vi "Host__Main.vi"() -> ()   [LabVIEW 2018]
doc: "Main program to be run from user pc for operating pod.\nMust be run before Master__Main.vi.\n\nContains an initialization section that forces the confirmation of system run parameters and sets variables to safe values. \nThere are 4 parallel loops for: GUI updates, user events, receiving data from target, sending data via UDP (per SpaceX's requirements)"
uses:
  Globals/Host_STOP.vi
  <vilib>/Utility/error.llb/DialogType.ctl
  Master/Control/TypeDef_DigitalOuts.ctl
  Master/Control/RunTypesLibrary/RunTypeList.ctl
  Master/TypeDef_RunParameters.ctl
  Globals/Host_RUNPARAMETERS.vi
  Libraries/TypeDef_ControlTabs.ctl
  Globals/Host_UDPGLOBALS.vi
  Type_Def/Master_DataControl.ctl
  Type_Def/TypeDef FixedMotorData.ctl
  Type_Def/Type_Def Actuator Controls.ctl
  Libraries/TypeDef_CurrentState.ctl
panel:
  out "Motor Target":dbl
  out "BMS Fault":bool
  out "BMS Connection":bool
  out "Low Side (BMS)":bool
  out "High Side (BMS)":bool
  out "Motor Fault":bool
  out "Ignition Indicator":bool caption="Ignition"
  out "Speed (mph)":dbl(graph)
  in  "ReIntCAN":bool
  in  "Acc Offset":bool
  in  "Reset Navigation":bool
  out "Pump Indicator":bool caption="Pump"
  in  "Dump Valve":bool
  out "Motor Controller State":u16(ring)=1 items=["unknown"=1, "boot-up"=0, "stopped"=4, "operational"=5, "pre-operational"=127, "connection lost"=128]
  out "Motor Alive":bool
  out "Distance (ft)":dbl
  out "Connected?":bool=TRUE
  out "UDP Sent":bool
  in  "DisableWatchdog":bool
  in  "Reset to Idle":bool
  in  "Manual Brake":bool
  out "Fault?":bool=TRUE
  out "Stripe Count":dbl
  out "24V Power Indicator":bool caption="Pod\nPower"
  out "Low Side Indicator":bool caption="Low\nSide"
  in  "DisableECheck":bool
  in  "Pod Power":bool
  out "HighSide Indicator":bool caption="High\nSide"
  out "Distance bar (ft)":dbl(slide) scale=0.0..5280.0 scale format="%.3f"
  out "Current State":T1
  in  "System Parameters":bool
  in  "Extended Details":bool
  in  "Save Data":bool
  out "Release Valve Indicator":bool caption="Dump\nValve"
  out "Current Time (ms)":dbl
  out "PrechargeIndicator":bool caption="Pre-\ncharge"
  out "Brakes Indicator":bool caption="Brakes"
  in  "Stop CRIO":bool
  in  "Simulate Data":bool
  out "Clamp Indicator":bool caption="Clamp"
  out "System Check Dialogue":string
  out "x Acceleration (g)":dbl(graph)
  out "HC Table":string[][](table) caption="Table Control"
  in  "ReInt Streams":bool
  in  "Stop Host":bool
  in  "Control Tab":T2=enum."Run"
  in  "Service Button (toggle)":bool
  in  "Service Button":bool
  in  "Drive Target (service)":i16 caption="Drive Target"
  in  "Drive Mode":enum16{"velocityMode", "torqueMode", ""}(ring)
  in  "driveEnable":bool
  in  "Ignition (service)":bool
  in  "Low Side (SC)":bool caption="Low\nSide"
  in  "HighSidePermission (SC)":bool caption="High\nSide"
  in  "Brakes (SC)":bool caption="Brakes"
  in  "Clamp (SC)":bool caption="Clamp"
  in  "HighSide (SC)":bool caption="High\nSide"
  in  "Precharge (SC)":bool caption="Pre-\nCharge"
  in  "Pump (SC)":bool caption="Pump"
  in  "Ignition (SC)":bool caption="Ignition"
  in  "Drive Enable (SC)":bool caption="Drive Enable"
  in  "Drive Mode (SC)":enum16{"velocityMode", "torqueMode", ""}(ring) caption="Drive Mode"
  in  "Drive Target (SC)":i16 caption="Drive Target"
  in  "Precharge":bool
  in  "Launch":bool
  in  "Ready":bool
  in  "Ignition":bool
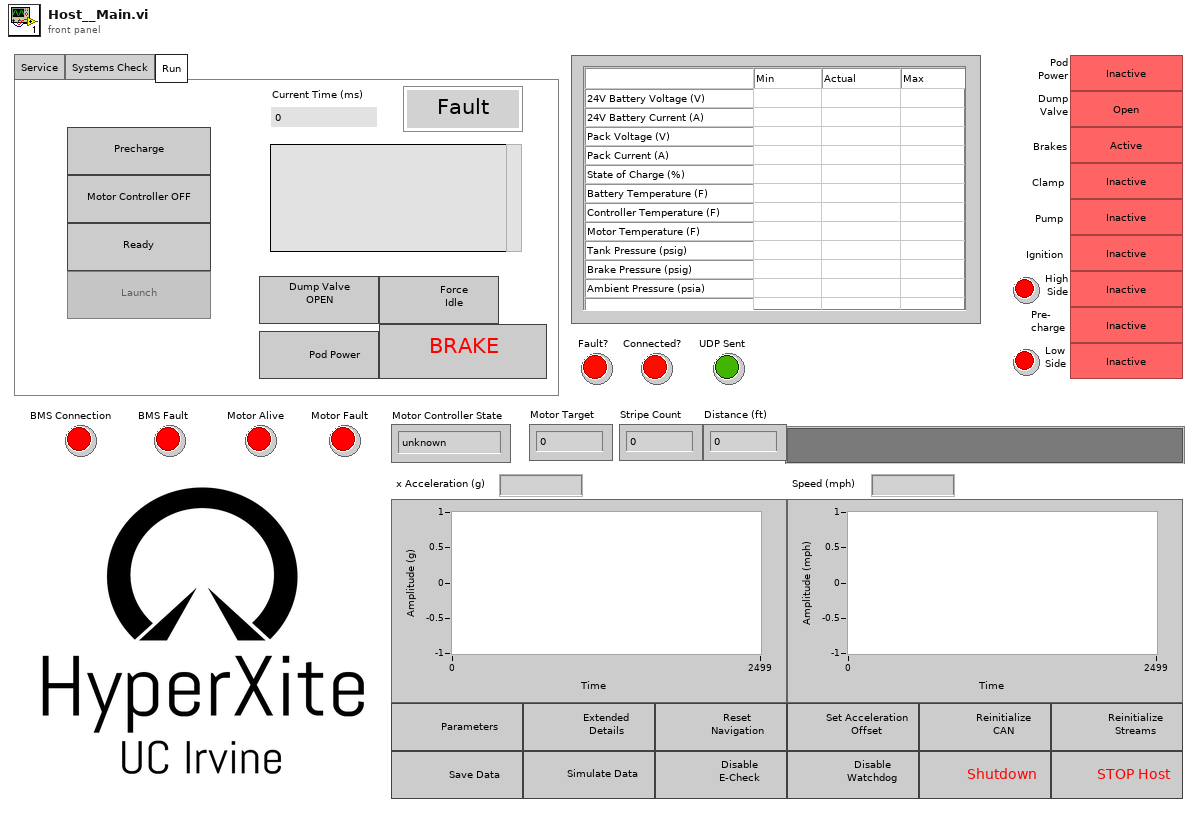
[diagram p1: front panel]
types:
  T1 = typedef "TypeDef_CurrentState.ctl" = enum16{"Fault", "Idle", "Ready", "Pushing", "Coast", "Braking"}
  T2 = typedef "TypeDef_ControlTabs.ctl" = enum32{"Service", "Systems Check", "Run"}
  T3 = typedef "DialogType.ctl" = u16
  T4 = enum8{"Enabled", "Disabled", "Disabled and Grayed Out"}
  T5 = typedef "RunTypeList.ctl" = enum16{"Full Run", "Systems Check", "Service"}
  T6 = typedef "TypeDef_RunParameters.ctl" = cluster{"Distance Threshold (ft)":dbl, "Time Threshold (s)":dbl, "Target (I16)":i16}
  T7 = typedef "TypeDef_DigitalOuts.ctl" = cluster{"Pod Power":bool, "Dump Valve":bool, "Brakes":bool, "Clamp":bool, "Pump":bool, "Ignition":bool, "DO6":bool, "DO7":bool, "HighSide":bool, "Precharge":bool, "LowSide":bool, "DO3":bool, "DO4":bool, "DO5":bool, "DO62":bool, "DO72":bool}
  T8 = typedef "Master_DataControl.ctl" = cluster{"cRIO Data":T9, "IMU Data":T10, "BMS Data":T11, "Motor Data":T13}
  T9 = typedef "TypeDef_cRIOData.ctl" = cluster{"HallEffect Right (cm)":dbl, "HallEffect Left (cm)":dbl, "Optical Sensor 1 (V)":dbl, "Optical Sensor 2 (V)":dbl, "24V Voltage  (V)":dbl, "24V Current (A)":dbl, "Contactor H1 Continuity":dbl, "Contactor L1 Continuity ":dbl, "Contactor H2 Continuity":dbl, "Contactor L2 Continuity ":dbl, "Brake PT(psig)":dbl, "Pump PT (psig)":dbl, "24V Temp   (C)":dbl, "Tank PT(psig) ":dbl, "ABS Pressure 1 (psig)":dbl, "ABS Pressure 2 (psig) ":dbl, "Displacement (ft)":dbl, "Velocity (ft/s)":dbl, "Time (ms)":dbl}
  T10 = typedef "Type_Def IMUData.ctl" = cluster{"x acceleration (g)":dbl, "Pressure (psia)":dbl, "Temperature (F)":dbl}
  T11 = typedef "TypeDef_BMSData.ctl" = cluster{"Pack 1 Max Cell\n Voltage (V)":dbl, "Pack 1 Max Cell\n ID ":dbl, "Pack 1 Min Cell \nVoltage (V)":dbl, "Pack 1 Min Cell \nID ":dbl, "Pack 1 State of Charge  (%)":dbl, "Pack 1 Average Voltage1 (V)":dbl, "Pack 1Voltage Delta (V)":dbl, "Pack 1 Current (A)":dbl, "Pack 1 Voltage (V)":dbl, "Pack 1 Max Resistance (Ohm)":dbl, "Pack 1Min Resistance (Ohm)":dbl, "Pack 1Average Resistance (Ohm)":dbl, "Pack 1Delta Resistance (Ohm)":dbl, "Pack 1 Highest Temperature(F)":dbl, "BmsStatus":T12, "Pack 2 Max Cell\n Voltage (V) ":dbl, "Pack 2 Max Cell\n ID  ":dbl, "Pack 2 Min Cell \nVoltage (V) ":dbl, "Pack 2 Min Cell \nID  ":dbl, "Pack 2 Average Voltage1 (V)":dbl, "Pack 2 Voltage Delta (V) ":dbl, "Pack 2 Current (A)":dbl, "Pack 2 Voltage (V) ":dbl, "Pack 2 State of Charge  (%) ":dbl, "Pack 2 Max Resistance (Ohm) ":dbl, "Pack 2 Min Resistance (Ohm)":dbl, "Pack 2 Average Resistance (Ohm)":dbl, "Pack 2 Delta Resistance (Ohm) ":dbl, "Pack 2 Highest Temperature(F) ":dbl}
  T12 = typedef "TypeDef_BmsStatus.ctl" = cluster{"Pack 1 Fault":bool, "Pack 1 Isolation":bool, "Pack  2 Fault":bool, "Pack 2 Isolation":bool}
  T13 = typedef "TypeDef FixedMotorData.ctl" = cluster{" Velocity (RPM)":dbl, " MotorTemp(C)":dbl, " ControlTemp(C)":dbl, " DcLinkVolt(V)":dbl, " ErrorCode":dbl, "IsAlive":bool, "motorStatus":cluster{"isReady":bool, "isOn":bool, "isOperEn":bool, "isFault":bool, "isVoltEn":bool, "targetReached":bool, "isWarning":bool}, "motorControllerState":u16}
  T14 = typedef "Type_Def Actuator Controls.ctl" = cluster{"Reverse ":bool, "Precharge Ctrl":bool, "Pump Ctrl":bool, "24 VDC Ctr":bool, "Vent Solenoid":bool, "Brake Solenoid":bool, "EMCY  Brake Solenoid":bool, "Digital Out 7B ":bool, "Forward Ctrl":bool, "Contact H1":bool, "Contact L1":bool, "Contact H2":bool, "Contact L2 ":bool, "LED RED":bool, "LED GREEN":bool, " Digital Out 7A":bool}
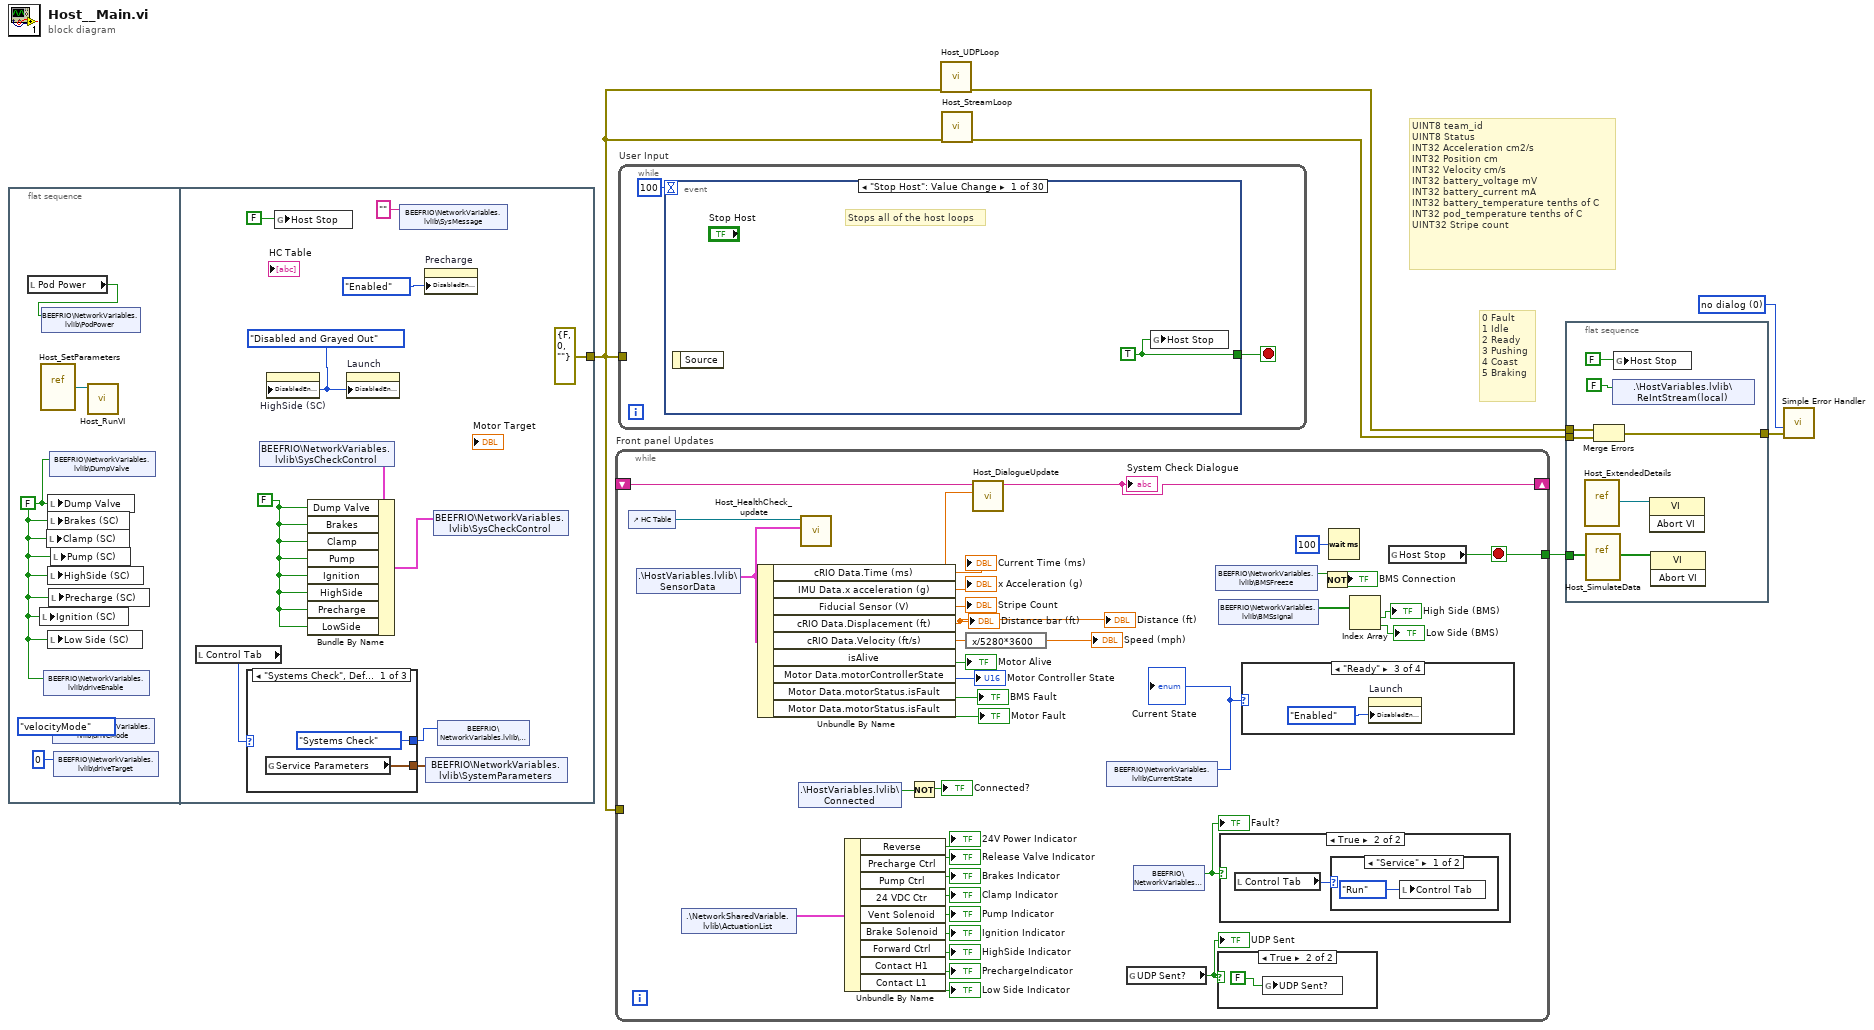
[diagram p0: block diagram]
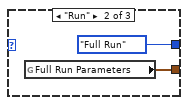
[diagram p2: hidden frame]
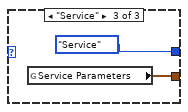
[diagram p3: hidden frame]
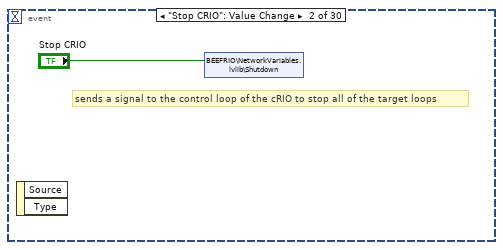
[diagram p4: hidden frame]
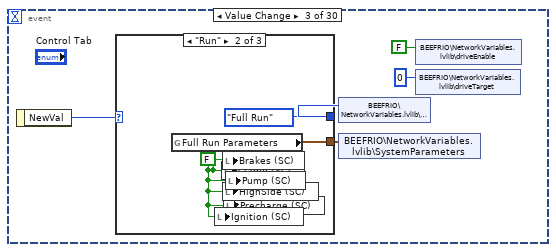
[diagram p5: hidden frame]
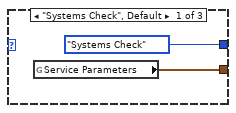
[diagram p6: hidden frame]
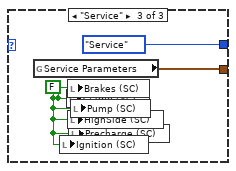
[diagram p7: hidden frame]
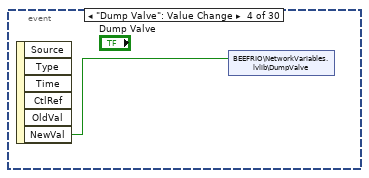
[diagram p8: hidden frame]
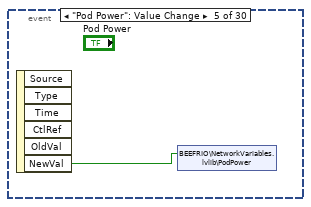
[diagram p9: hidden frame]
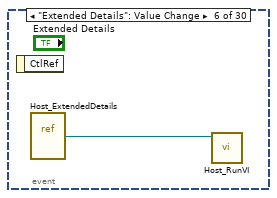
[diagram p10: hidden frame]
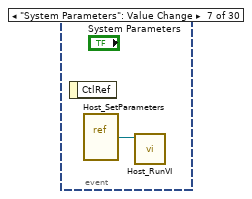
[diagram p11: hidden frame]
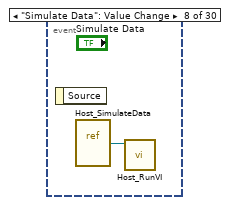
[diagram p12: hidden frame]
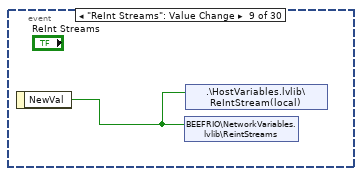
[diagram p13: hidden frame]
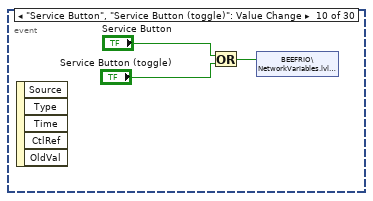
[diagram p14: hidden frame]
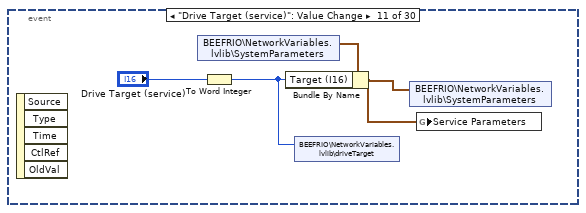
[diagram p15: hidden frame]
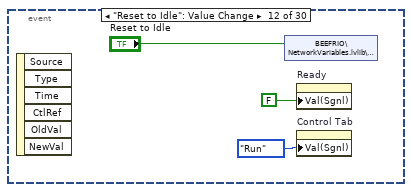
[diagram p16: hidden frame]
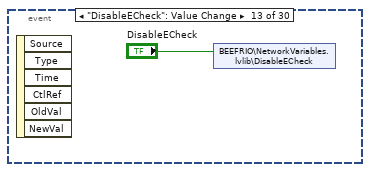
[diagram p17: hidden frame]
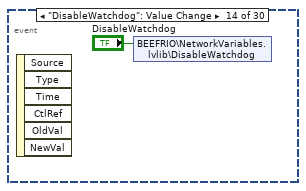
[diagram p18: hidden frame]
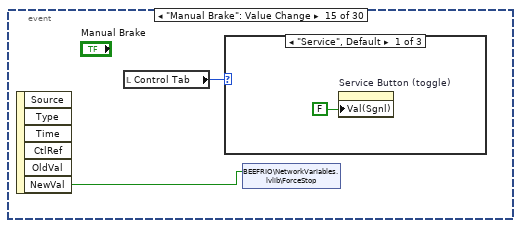
[diagram p19: hidden frame]
diagram:
  w3 = T3 0 items=["no dialog", "OK message", "continue or stop message", "OK message + warnings", "continue/stop + warnings"] ("type of dialog (OK msg:1)")
  # "0 Fault\n1 Idle\n2 Ready\n3 Pushing\n4 Coast\n5 Braking"
  # "UINT8 team_id\nUINT8 Status\nINT32 Acceleration cm2/s\nINT32 Position cm\nINT32 Velocity cm/s\nINT32 battery_voltage mV\nINT32 battery_current mA\nINT32 battery_temperature tenths of C\nINT32 pod_temperature tenths of C\nUINT32 Stripe count"
  n1 = flat-sequence {
    tunnel: [errorcluster {"status"=FALSE, "code"=0, "source"=""} ("error IO")] -> w1
    frame #0 {
      w9 = FALSE ("Dump Valve")
      n2 = local read "Pod Power"() -> (w10:bool)
      n3 = local write "Ignition (SC)"(w9) -> ()
      n4 = vi-ref "Host_SetParameters.vi"() -> (w11:refnum<vi>)
      n5 = shared-variable "BEEFRIO\\NetworkVariables.lvlib\\PodPower"(w10) -> ()  [unwired: 1 in, 1 out]
      n6 = shared-variable "BEEFRIO\\NetworkVariables.lvlib\\driveEnable"(w9) -> ()  [unwired: 1 in, 1 out]
      n7 = local write "Clamp (SC)"(w9) -> ()
      n8 = local write "Dump Valve"(w9) -> ()
      n9 = local write "Brakes (SC)"(w9) -> ()
      n10 = local write "HighSide (SC)"(w9) -> ()
      n11 = local write "Low Side (SC)"(w9) -> ()
      n12 = local write "Precharge (SC)"(w9) -> ()
      n13 = shared-variable "BEEFRIO\\NetworkVariables.lvlib\\DumpValve"(w9) -> ()  [unwired: 1 in, 1 out]
      n14 = local write "Pump (SC)"(w9) -> ()
      n15 = shared-variable "BEEFRIO\\NetworkVariables.lvlib\\driveMode"(enum16{"velocityMode", "torqueMode", ""}."velocityMode" ("driveMode")) -> ()  [unwired: 1 in, 1 out]
      n16 = shared-variable "BEEFRIO\\NetworkVariables.lvlib\\driveTarget"(i16 0 ("driveTarget")) -> ()  [unwired: 1 in, 1 out]
      n17 = call "Host_RunVI.vi"("VI in"=w11) -> ()  [unwired: 11 in]
    }
    frame #1 {
      w14 = T4."Disabled and Grayed Out" ("Disabled")
      w13 = FALSE ("Actuators.Dump Valve")
      n18 = local read "Control Tab"() -> (w20:T2)
      n19 = case shown="\"Systems Check\", Default" w20 {
        tunnel: [RunTypeList."Systems Check" ("t") RunTypeList."Full Run" ("RunType") RunTypeList."Service" ("t")] -> w19
        tunnel: [w23 w25 w28] -> w18
        frame "Systems Check", Default {
          n20 = global read "Host_RUNPARAMETERS.vi" "Service Parameters"() -> (w23:T6)
        }
        frame "Run" {
          n21 = global read "Host_RUNPARAMETERS.vi" "Full Run Parameters"() -> (w25:T6)
        }
        frame "Service" {
          n22 = global read "Host_RUNPARAMETERS.vi" "Service Parameters"() -> (w28:T6)
        }
      }
      n23 = shared-variable "BEEFRIO\\NetworkVariables.lvlib\\SysCheckControl"() -> (w17:T7)  [unwired: 1 in, 1 out]
      n24 = property on="HighSide (SC)" class="Bool (strict)"("DisabledEnum"=w14) -> ()  [unwired: 2 in, 2 out]
      n25 = global write "Host_STOP.vi" "Host Stop"(FALSE ("StopControl")) -> ()
      n26 = Bundle By Name(cluster=w17, "Dump Valve"=w13, "Brakes"=w13, "Clamp"=w13, "Pump"=w13, "Ignition"=w13, "HighSide"=w13, "Precharge"=w13, "LowSide"=w13) -> (w16:T7)
      n27 = property on="Launch" class="Bool"("DisabledEnum"=w14) -> ()  [unwired: 2 in, 2 out]
      n28 = shared-variable "BEEFRIO\\NetworkVariables.lvlib\\SysMessage"("" ("SysMessage")) -> ()  [unwired: 1 in, 1 out]
      n29 = property on="Precharge" class="Bool"("DisabledEnum"=T4."Enabled" ("Disabled")) -> ()  [unwired: 2 in, 2 out]
      n30 = shared-variable "BEEFRIO\\NetworkVariables.lvlib\\SystemParameters"(w18) -> ()  [unwired: 1 in, 1 out]
      n31 = shared-variable "BEEFRIO\\NetworkVariables.lvlib\\SysCheckControl"(w16) -> ()  [unwired: 1 in, 1 out]
      n32 = shared-variable "BEEFRIO\\NetworkVariables.lvlib\\RunType"(w19) -> ()  [unwired: 1 in, 1 out]
    }
  }
  n33 = while "Front panel Updates" {
    tunnel: [w63] -> w5
    shift-right: [w61] -> _
    shift-left: _ -> [w62]
    tunnel: w1 -> [_]
    stop <- w63 stop-if-true
    n34 = control-ref of="HC Table"() -> (w59:refnum<vi>)
    n35 = shared-variable ".\\HostVariables.lvlib\\SensorData"() -> (w58:T8)  [unwired: 1 in, 1 out]
    n36 = shared-variable ".\\NetworkSharedVariable.lvlib\\ActuationList"() -> (w60:T14)  [unwired: 1 in, 1 out]
    n37 = Unbundle By Name(w58) -> ("cRIO Data.Time (ms)"=w55:dbl, "IMU Data.x acceleration (g)"=→"x Acceleration (g)":dbl, "Fiducial Sensor (V)"=→"Stripe Count":dbl, "cRIO Data.Displacement (ft)"=→"Distance bar (ft)" →"Distance (ft)":dbl, "cRIO Data.Velocity (ft/s)"=w51:dbl, "isAlive"=→"Motor Alive":bool, "Motor Data.motorControllerState"=→"Motor Controller State":u16, "Motor Data.motorStatus.isFault"=→"BMS Fault":bool, "Motor Data.motorStatus.isFault"=→"Motor Fault":bool)
    "Current Time (ms)" <- w55
    n38 = shared-variable ".\\HostVariables.lvlib\\Connected"() -> (w53:bool)  [unwired: 1 in, 1 out]
    n39 = call "Host_HealthCheck_update.vi"("reference in"=w59, "input cluster"=w58) -> ()  [unwired: 9 in]
    n40 = Unbundle By Name(w60) -> ("Reverse"=→"24V Power Indicator":bool, "Precharge Ctrl"=→"Release Valve Indicator":bool, "Pump Ctrl"=→"Brakes Indicator":bool, "24 VDC Ctr"=→"Clamp Indicator":bool, "Vent Solenoid"=→"Pump Indicator":bool, "Brake Solenoid"=→"Ignition Indicator":bool, "Forward Ctrl"=→"HighSide Indicator":bool, "Contact H1"=→"PrechargeIndicator":bool, "Contact L1"=→"Low Side Indicator":bool)
    n41 = Not(x=w53) -> (.not. x?=→"Connected?":bool)
    n42 = expression code="x/5280*3600"(w51) -> (→"Speed (mph)":dbl)
    n43 = call "Host_DialogueUpdate.vi"("Time in"=w55, "String in"=w62) -> ("String out"=w61:string)  [unwired: 9 in]
    "System Check Dialogue" <- w61
    n44 = shared-variable "BEEFRIO\\NetworkVariables.lvlib\\CurrentState"() -> (w57:T1)  [unwired: 1 in, 1 out]
    "Current State" <- w57
    n45 = global read "Host_UDPGLOBALS.vi" "UDP Sent?"() -> (w49:bool)
    "UDP Sent" <- w49
    n46 = shared-variable "BEEFRIO\\NetworkVariables.lvlib\\Fault"() -> (w46:bool)  [unwired: 1 in, 1 out]
    "Fault?" <- w46
    n47 = shared-variable "BEEFRIO\\NetworkVariables.lvlib\\BMSFreeze"() -> (w34:bool)  [unwired: 1 in, 1 out]
    n48 = case shown="True" w49 {
      frame False {
      }
      frame True {
        n49 = global write "Host_UDPGLOBALS.vi" "UDP Sent?"(FALSE ("UDPSent?")) -> ()
      }
    }
    n50 = shared-variable "BEEFRIO\\NetworkVariables.lvlib\\BMSsignal"() -> (w35:bool[])  [unwired: 1 in, 1 out]
    n51 = case shown="True" w46 {
      frame False {
      }
      frame True {
        n52 = local read "Control Tab"() -> (w65:T2)
        n53 = case shown="\"Service\"" w65 {
          frame "Service" {
            n54 = local write "Control Tab"(TypeDef_ControlTabs."Run" ("Control Tab")) -> ()
          }
          frame Default {
          }
        }
      }
    }
    n55 = case shown="\"Ready\"" w57 {
      frame Default {
      }
      frame "Idle" {
        n56 = property on="Launch" class="Bool"("DisabledEnum"=T4."Disabled and Grayed Out" ("Disabled")) -> ()  [unwired: 2 in, 2 out]
      }
      frame "Ready" {
        n57 = property on="Launch" class="Bool"("DisabledEnum"=T4."Enabled" ("Disabled")) -> ()  [unwired: 2 in, 2 out]
      }
      frame "Pushing" {
        n58 = property on="Launch" class="Bool"("DisabledEnum"=T4."Disabled and Grayed Out" ("Disabled")) -> ()  [unwired: 2 in, 2 out]
      }
    }
    n59 = Not(x=w34) -> (.not. x?=→"BMS Connection":bool)
    n60 = Wait (ms)(milliseconds to wait=u32 100) -> ()  [unwired: 1 out]
    n61 = Index Array(array=w35) -> (element #1=→"High Side (BMS)":bool, element #2=→"Low Side (BMS)":bool)  [unwired: 2 in]
    n62 = global read "Host_STOP.vi" "Host Stop"() -> (w63:bool)
  }
  n63 = while "User Input" {
    tunnel: w1 -> [_]
    stop <- w72 stop-if-true
    n64 = event shown="[0] \"Stop Host\": Value Change" {
      selector: _ -> [_ _ _ _ _ _ _ _ _ _ _ _ _ _ _ _ _ _ _ _ _ _ _ _ _ _ _ _ _ _]
      dyn-events: _ -> [_ _ _ _ _ _ _ _ _ _ _ _ _ _ _ _ _ _ _ _ _ _ _ _ _ _ _ _ _ _]
      timeout: 100 -> [_ _ _ _ _ _ _ _ _ _ _ _ _ _ _ _ _ _ _ _ _ _ _ _ _ _ _ _ _ _]
      tunnel: [w73 _ _ _ _ _ _ _ _ _ _ _ _ _ _ _ FALSE ("element") FALSE ("element") FALSE ("element") _ _ _ _ _ _ _ _ _ _ _] -> w72
      event "Stop Host": Value Change {
        w73 = TRUE ("element")
        # "Stops all of the host loops"
        n65 = event-data() -> ()  [unwired: 1 in, 1 out]
        n66 = global write "Host_STOP.vi" "Host Stop"(w73) -> ()
      }
      event "Stop CRIO": Value Change {
        # "sends a signal to the control loop of the cRIO to stop all of the target loops"
        n67 = event-data() -> ()  [unwired: 1 in, 2 out]
        n68 = shared-variable "BEEFRIO\\NetworkVariables.lvlib\\Shutdown"("Stop CRIO") -> ()  [unwired: 1 in, 1 out]
      }
      event Value Change {
        n69 = event-data() -> ("NewVal"=w78:T2)  [unwired: 1 in]
        n70 = case shown="\"Run\"" w78 {
          tunnel: [RunTypeList."Systems Check" ("t") RunTypeList."Full Run" ("RunType") RunTypeList."Service" ("t")] -> w79
          tunnel: [w80 w83 w86] -> w77
          frame "Systems Check", Default {
            n71 = global read "Host_RUNPARAMETERS.vi" "Service Parameters"() -> (w80:T6)
          }
          frame "Run" {
            w82 = FALSE ("Dump Valve")
            n72 = global read "Host_RUNPARAMETERS.vi" "Full Run Parameters"() -> (w83:T6)
            n73 = local write "Ignition (SC)"(w82) -> ()
            n74 = local write "Clamp (SC)"(w82) -> ()
            n75 = local write "Brakes (SC)"(w82) -> ()
            n76 = local write "HighSide (SC)"(w82) -> ()
            n77 = local write "Precharge (SC)"(w82) -> ()
            n78 = local write "Pump (SC)"(w82) -> ()
          }
          frame "Service" {
            w85 = FALSE ("Dump Valve")
            n79 = global read "Host_RUNPARAMETERS.vi" "Service Parameters"() -> (w86:T6)
            n80 = local write "Ignition (SC)"(w85) -> ()
            n81 = local write "Clamp (SC)"(w85) -> ()
            n82 = local write "Brakes (SC)"(w85) -> ()
            n83 = local write "HighSide (SC)"(w85) -> ()
            n84 = local write "Precharge (SC)"(w85) -> ()
            n85 = local write "Pump (SC)"(w85) -> ()
          }
        }
        n86 = shared-variable "BEEFRIO\\NetworkVariables.lvlib\\RunType"(w79) -> ()  [unwired: 1 in, 1 out]
        n87 = shared-variable "BEEFRIO\\NetworkVariables.lvlib\\SystemParameters"(w77) -> ()  [unwired: 1 in, 1 out]
        n88 = shared-variable "BEEFRIO\\NetworkVariables.lvlib\\driveEnable"(FALSE ("driveEnable")) -> ()  [unwired: 1 in, 1 out]
        n89 = shared-variable "BEEFRIO\\NetworkVariables.lvlib\\driveTarget"(i16 0 ("driveTarget")) -> ()  [unwired: 1 in, 1 out]
      }
      event "Dump Valve": Value Change {
        n90 = event-data() -> ("NewVal"=w88:bool)  [unwired: 1 in, 5 out]
        n91 = shared-variable "BEEFRIO\\NetworkVariables.lvlib\\DumpValve"(w88) -> ()  [unwired: 1 in, 1 out]
      }
      event "Pod Power": Value Change {
        n92 = event-data() -> ("NewVal"=w89:bool)  [unwired: 1 in, 5 out]
        n93 = shared-variable "BEEFRIO\\NetworkVariables.lvlib\\PodPower"(w89) -> ()  [unwired: 1 in, 1 out]
      }
      event "Extended Details": Value Change {
        n94 = event-data() -> ()  [unwired: 1 in, 1 out]
        n95 = vi-ref "Host_ExtendedDetails.vi"() -> (w90:refnum<vi>)
        n96 = call "Host_RunVI.vi"("VI in"=w90) -> ()  [unwired: 11 in]
      }
      event "System Parameters": Value Change {
        n97 = event-data() -> ()  [unwired: 1 in, 1 out]
        n98 = vi-ref "Host_SetParameters.vi"() -> (w91:refnum<vi>)
        n99 = call "Host_RunVI.vi"("VI in"=w91) -> ()  [unwired: 11 in]
      }
      event "Simulate Data": Value Change {
        n100 = event-data() -> ()  [unwired: 1 in, 1 out]
        n101 = vi-ref "Host_SimulateData.vi"() -> (w92:refnum<vi>)
        n102 = call "Host_RunVI.vi"("VI in"=w92) -> ()  [unwired: 11 in]
      }
      event "ReInt Streams": Value Change {
        n103 = event-data() -> ("NewVal"=w93:bool)  [unwired: 1 in]
        n104 = shared-variable "BEEFRIO\\NetworkVariables.lvlib\\ReintStreams"(w93) -> ()  [unwired: 1 in, 1 out]
        n105 = shared-variable ".\\HostVariables.lvlib\\ReIntStream(local)"(w93) -> ()  [unwired: 1 in, 1 out]
      }
      event "Service Button", "Service Button (toggle)": Value Change {
        n106 = event-data() -> ()  [unwired: 1 in, 5 out]
        n107 = Or(x="Service Button", y="Service Button (toggle)") -> (x .or. y?=w94:bool)
        n108 = shared-variable "BEEFRIO\\NetworkVariables.lvlib\\Service"(w94) -> ()  [unwired: 1 in, 1 out]
      }
      event "Drive Target (service)": Value Change {
        n109 = event-data() -> ()  [unwired: 1 in, 5 out]
        n110 = shared-variable "BEEFRIO\\NetworkVariables.lvlib\\SystemParameters"() -> (w100:T6)  [unwired: 1 in, 1 out]
        n111 = To Word Integer(number="Drive Target (service)") -> (16bit integer=w97:i16)
        n112 = Bundle By Name(cluster=w100, "Target (I16)"=w97) -> (w99:T6)
        n113 = shared-variable "BEEFRIO\\NetworkVariables.lvlib\\driveTarget"(w97) -> ()  [unwired: 1 in, 1 out]
        n114 = shared-variable "BEEFRIO\\NetworkVariables.lvlib\\SystemParameters"(w99) -> ()  [unwired: 1 in, 1 out]
        n115 = global write "Host_RUNPARAMETERS.vi" "Service Parameters"(w99) -> ()
      }
      event "Reset to Idle": Value Change {
        n116 = event-data() -> ()  [unwired: 1 in, 6 out]
        n117 = shared-variable "BEEFRIO\\NetworkVariables.lvlib\\ForceIdle"("Reset to Idle") -> ()  [unwired: 1 in, 1 out]
        n118 = property on="Ready" class="Bool (strict)"("Val(Sgnl)"=FALSE ("Ready")) -> ()  [unwired: 2 in, 2 out]
        n119 = property on="Control Tab" class="TabCtl (strict)"("Val(Sgnl)"=TypeDef_ControlTabs."Run" ("Value (Signaling)")) -> ()  [unwired: 2 in, 2 out]
      }
      event "DisableECheck": Value Change {
        n120 = event-data() -> ()  [unwired: 1 in, 6 out]
        n121 = shared-variable "BEEFRIO\\NetworkVariables.lvlib\\DisableECheck"("DisableECheck") -> ()  [unwired: 1 in, 1 out]
      }
      event "DisableWatchdog": Value Change {
        n122 = event-data() -> ()  [unwired: 1 in, 6 out]
        n123 = shared-variable "BEEFRIO\\NetworkVariables.lvlib\\DisableWatchdog"("DisableWatchdog") -> ()  [unwired: 1 in, 1 out]
      }
      event "Manual Brake": Value Change {
        n124 = event-data() -> ("NewVal"=w107:bool)  [unwired: 1 in, 5 out]
        n125 = local read "Control Tab"() -> (w106:T2)
        n126 = case shown="\"Service\", Default" w106 {
          frame "Service", Default {
            n127 = property on="Service Button (toggle)" class="Bool (strict)"("Val(Sgnl)"=FALSE ("Value (Signaling)")) -> ()  [unwired: 2 in, 2 out]
          }
          frame "Systems Check" {
          }
          frame "Run" {
          }
        }
        n128 = shared-variable "BEEFRIO\\NetworkVariables.lvlib\\ForceStop"(w107) -> ()  [unwired: 1 in, 1 out]
      }
      event "Ready": Value Change {
        n129 = event-data() -> ("NewVal"=w109:bool)  [unwired: 1 in, 5 out]
        n130 = shared-variable "BEEFRIO\\NetworkVariables.lvlib\\Ready"(w109) -> ()  [unwired: 1 in, 1 out]
      }
      event "Precharge (SC)": Value Change {
        n131 = event-data() -> ()  [unwired: 1 in, 6 out]
        n132 = shared-variable "BEEFRIO\\NetworkVariables.lvlib\\SysCheckControl"() -> (w115:T7)  [unwired: 1 in, 1 out]
        n133 = local read "HighSidePermission (SC)"() -> (w112:bool)
        n134 = Bundle By Name(cluster=w115, "Precharge"="Precharge (SC)") -> (w116:T7)
        n135 = Or(x="Precharge (SC)", y=w112) -> (x .or. y?=w111:bool)
        n136 = shared-variable "BEEFRIO\\NetworkVariables.lvlib\\SysCheckControl"(w116) -> ()  [unwired: 1 in, 1 out]
        n137 = Select(t=T4."Enabled" ("Disabled"), s=w111, f=T4."Disabled and Grayed Out" ("Disabled")) -> (s? t:f=w114:T4)
        n138 = property on="HighSide (SC)" class="Bool (strict)"("DisabledEnum"=w114) -> ()  [unwired: 2 in, 2 out]
      }
      event "HighSidePermission (SC)": Value Change {
        n139 = event-data() -> ()  [unwired: 1 in, 6 out]
        n140 = Select(t=T4."Enabled" ("Disabled"), s="HighSidePermission (SC)", f=T4."Disabled and Grayed Out" ("Disabled")) -> (s? t:f=w123:T4)
        n141 = property on="HighSide (SC)" class="Bool (strict)"("DisabledEnum"=w123) -> ()  [unwired: 2 in, 2 out]
      }
      event "HighSide (SC)": Value Change {
        n142 = event-data() -> ()  [unwired: 1 in, 6 out]
        n143 = control-ref of="Precharge (SC)"() -> (w129:refnum<vi>)
        n144 = property class="Bool (strict)"(reference=w129) -> (reference out=w127:refnum<vi>, "Value"=w128:bool)  [unwired: 1 in, 1 out]
        n145 = shared-variable "BEEFRIO\\NetworkVariables.lvlib\\SysCheckControl"() -> (w131:T7)  [unwired: 1 in, 1 out]
        n146 = Bundle By Name(cluster=w131, "HighSide"="HighSide (SC)") -> (w126:T7)
        n147 = case shown="True" w128 {
          tunnel: w127 -> [_ w137]
          tunnel: w126 -> [w132 w135]
          tunnel: [w132 w134] -> w125
          frame False {
          }
          frame True {
            n148 = property class="Bool (strict)"(reference=w137, "Value"=FALSE) -> ()  [unwired: 1 in, 2 out]
            n149 = Bundle By Name(cluster=w135, "Precharge"=FALSE ("Actuators.PrechargeContactor")) -> (w134:T7)
          }
        }
        n150 = shared-variable "BEEFRIO\\NetworkVariables.lvlib\\SysCheckControl"(w125) -> ()  [unwired: 1 in, 1 out]
      }
      event "Clamp (SC)", "Brakes (SC)", "Pump (SC)", "Ignition (SC)", "Low Side (SC)": Value Change {
        n151 = event-data() -> ()  [unwired: 1 in, 1 out]
        n152 = shared-variable "BEEFRIO\\NetworkVariables.lvlib\\SysCheckControl"() -> (w143:T7)  [unwired: 1 in, 1 out]
        n153 = Bundle By Name(cluster=w143, "Brakes"="Brakes (SC)", "Clamp"="Clamp (SC)", "Pump"="Pump (SC)", "Ignition"="Ignition (SC)", "LowSide"="Low Side (SC)") -> (w144:T7)
        n154 = shared-variable "BEEFRIO\\NetworkVariables.lvlib\\SysCheckControl"(w144) -> ()  [unwired: 1 in, 1 out]
      }
      event "Ignition": Value Change {
        n155 = event-data() -> ()  [unwired: 1 in, 1 out]
        n156 = Or(x="Ignition", y="Ignition (service)") -> (x .or. y?=w146:bool)
        n157 = shared-variable "BEEFRIO\\NetworkVariables.lvlib\\Ignition"(w146) -> ()  [unwired: 1 in, 1 out]
      }
      event "Drive Enable (SC)", "Drive Mode (SC)", "Drive Target (SC)": Value Change {
        n158 = event-data() -> ()  [unwired: 1 in, 1 out]
        n159 = shared-variable "BEEFRIO\\NetworkVariables.lvlib\\driveEnable"("Drive Enable (SC)") -> ()  [unwired: 1 in, 1 out]
        n160 = shared-variable "BEEFRIO\\NetworkVariables.lvlib\\driveMode"("Drive Mode (SC)") -> ()  [unwired: 1 in, 1 out]
        n161 = shared-variable "BEEFRIO\\NetworkVariables.lvlib\\driveTarget"("Drive Target (SC)") -> ()  [unwired: 1 in, 1 out]
      }
      event "Launch": Value Change {
        n162 = event-data() -> ("NewVal"=w152:bool)  [unwired: 1 in]
        n163 = shared-variable "BEEFRIO\\NetworkVariables.lvlib\\Launch"(w152) -> ()  [unwired: 1 in, 1 out]
        n164 = local write "Ready"(FALSE ("Ready")) -> ()
      }
      event "Precharge": Value Change {
        n165 = event-data() -> ()  [unwired: 1 in, 2 out]
        n166 = shared-variable "BEEFRIO\\NetworkVariables.lvlib\\Precharge"("Precharge") -> ()  [unwired: 1 in, 1 out]
      }
      event "driveEnable", "Drive Mode": Value Change {
        n167 = event-data() -> ()  [unwired: 1 in, 2 out]
        n168 = shared-variable "BEEFRIO\\NetworkVariables.lvlib\\driveMode"("Drive Mode") -> ()  [unwired: 1 in, 1 out]
        n169 = shared-variable "BEEFRIO\\NetworkVariables.lvlib\\driveEnable"("driveEnable") -> ()  [unwired: 1 in, 1 out]
      }
      event "Reset Navigation": Value Change {
        n170 = event-data() -> ()  [unwired: 1 in, 2 out]
        n171 = shared-variable "BEEFRIO\\NetworkVariables.lvlib\\NavReset"("Reset Navigation") -> ()  [unwired: 1 in, 1 out]
      }
      event "Acc Offset": Value Change {
        n172 = event-data() -> ()  [unwired: 1 in, 2 out]
        n173 = shared-variable "BEEFRIO\\NetworkVariables.lvlib\\CalcAccelerationOffset"("Acc Offset") -> ()  [unwired: 1 in, 1 out]
      }
      event "ReIntCAN": Value Change {
        n174 = event-data() -> ()  [unwired: 1 in, 2 out]
        n175 = shared-variable "BEEFRIO\\NetworkVariables.lvlib\\ReintCAN"("ReIntCAN") -> ()  [unwired: 1 in, 1 out]
      }
      event Timeout {
        n176 = event-data() -> ()  [unwired: 1 in, 1 out]
      }
      event "Save Data": Value Change {
        n177 = event-data() -> ()  [unwired: 1 in, 1 out]
        n178 = vi-ref "Host_SaveToFile.vi"() -> (w159:refnum<vi>)
        n179 = call "Host_RunVI.vi"("VI in"=w159) -> ()  [unwired: 11 in]
      }
    }
  }
  n180 = call "Host_UDPLoop.vi"("error in (no error)"=w1) -> ("error out"=w4:errorcluster)  [unwired: 10 in]
  n181 = call "Host_StreamLoop.vi"("error in (no error)"=w1) -> ("error out"=w6:errorcluster)  [unwired: 10 in]
  n182 = flat-sequence {
    tunnel: w6 -> [w164]
    tunnel: w5 -> [_]
    tunnel: w4 -> [w163]
    tunnel: [w162] -> w2
    frame #0 {
      n183 = vi-ref "Host_ExtendedDetails.vi"() -> (w165:refnum<vi>)
      n184 = vi-ref "Host_SimulateData.vi"() -> (w161:refnum<vi>)
      n185 = Merge Errors(w163, w164) -> (w162:errorcluster)
      n186 = shared-variable ".\\HostVariables.lvlib\\ReIntStream(local)"(FALSE ("ReInt Stream")) -> ()  [unwired: 1 in, 1 out]
      n187 = global write "Host_STOP.vi" "Host Stop"(FALSE ("StopControl")) -> ()
      n188 = invoke class="VI" method="Abort VI"(reference=w165) -> ()  [unwired: 2 in, 3 out]
      n189 = invoke class="VI" method="Abort VI"(reference=w161) -> ()  [unwired: 2 in, 3 out]
    }
  }
  n190 = call <vilib>:"Simple Error Handler.vi"("type of dialog (OK msg:1)"=w3, "error in (no error)"=w2) -> ()  [unwired: 3 in, 5 out]
